vi "test_resist_last.vi"() -> ()   [LabVIEW 2015]
uses:
  global_qaqc.vi
panel:
  out "Output file path":path
  out "Name of PCB":string
  in  "Redo":bool
  out "Last value (MOhm)":dbl
  out "Boolean 16":bool
  out "Boolean 15":bool
  out "Boolean 14":bool
  out "Boolean 13":bool
  out "Boolean 12":bool
  out "Boolean 11":bool
  out "Boolean 10":bool
  out "Boolean 9":bool
  out "Boolean 8":bool
  out "Boolean 7":bool
  out "Boolean 6":bool
  out "Boolean 5":bool
  out "Boolean 4":bool
  out "Boolean 3":bool
  out "Boolean 2":bool
  out "Boolean":bool
  in  "Open Database":bool
  in  "Close VI":bool
  in  "?":bool
  # "Electrometer Test"
  # "1) Setup the measure and then click \"Acquire\". If you want to take again the last measure, click \"Redo last\" and then \"Acquire\""
  # "Yellow: Done"
  # "Green: OK"
  # "Yellow: Done"
  # "Green: OK"
  # "Circular small LED \n\nGREY --> Measure NOT DONE\nYELLOW --> Measure DONE\n\n\nElliptic big LED\n\nRED --> Value not taken OR out of range\nGREEN --> Value in range"
  # "2) Once measure is finished, open the database and upload the file"
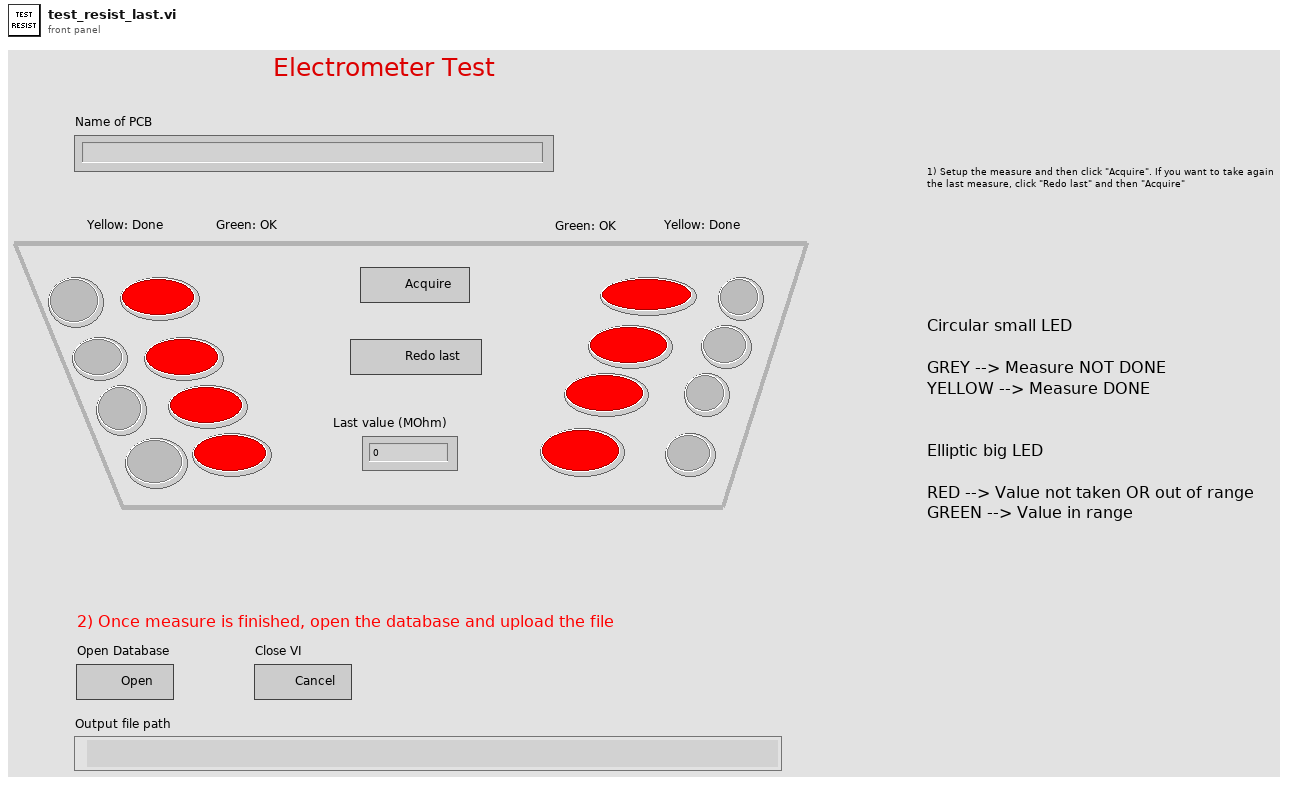
[diagram p1: front panel]
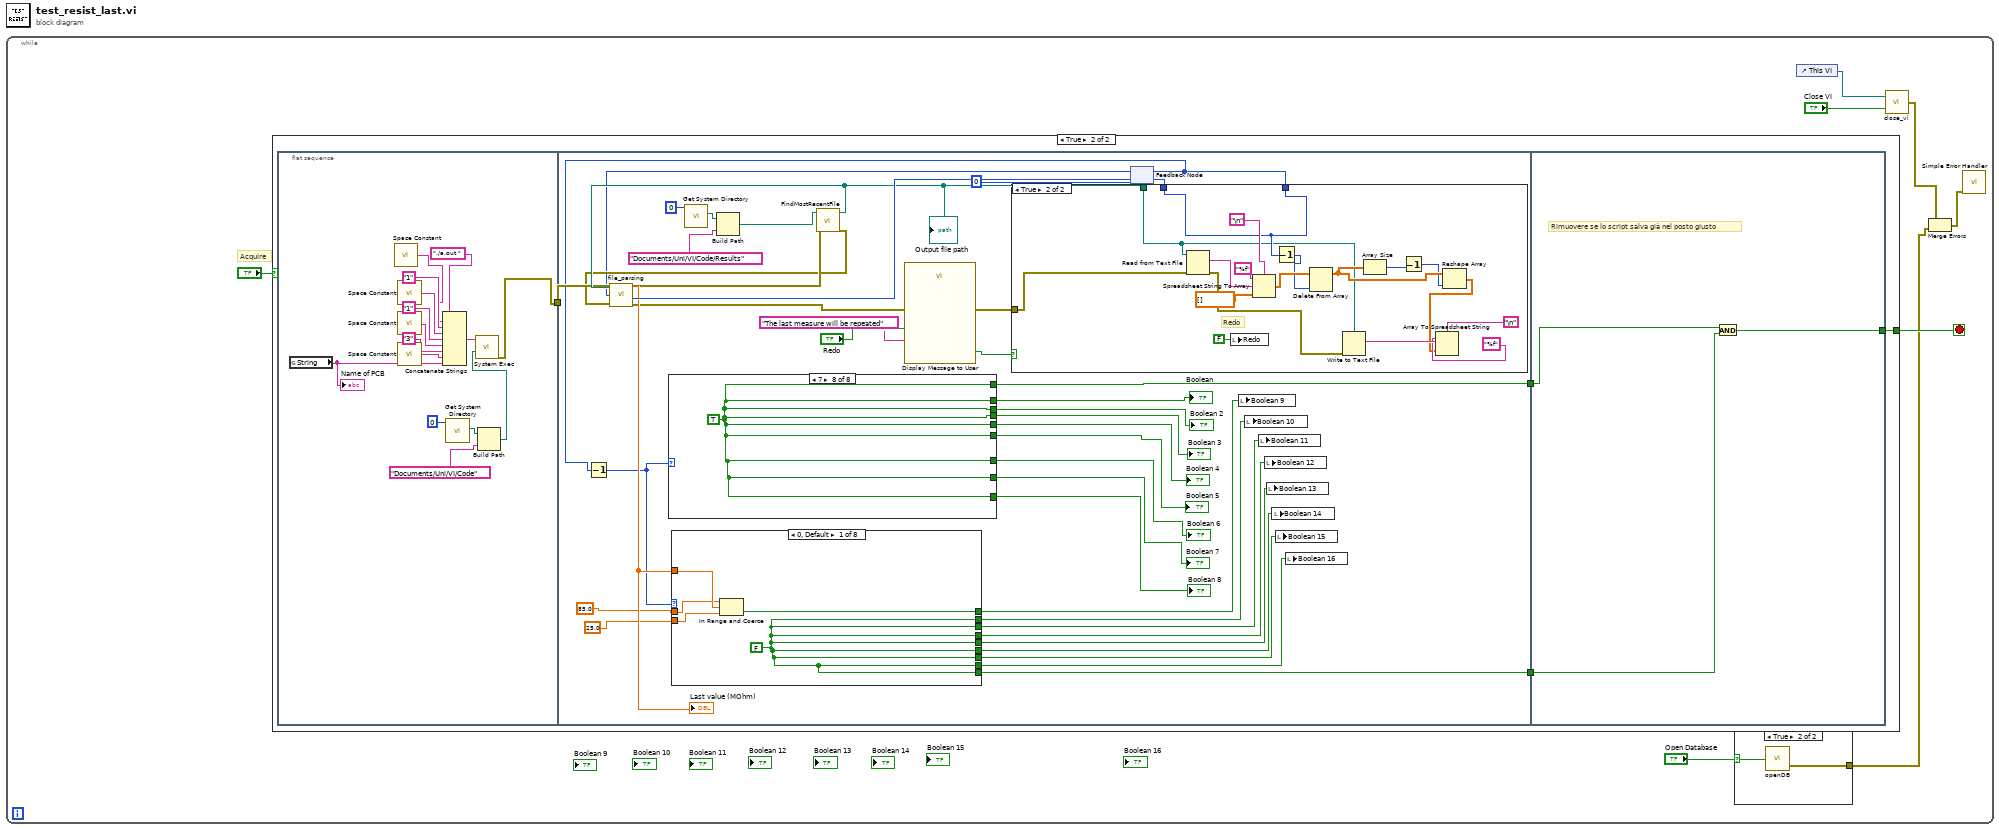
[diagram p0: block diagram]
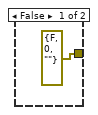
[diagram p2: hidden frame]
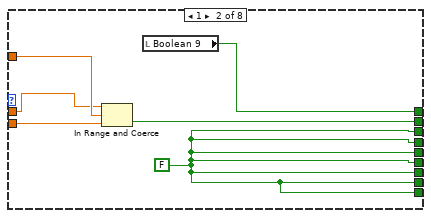
[diagram p4: hidden frame]
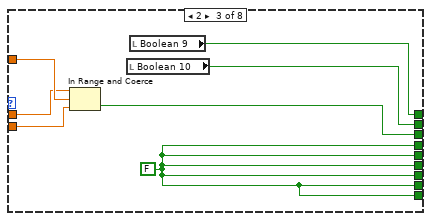
[diagram p5: hidden frame]
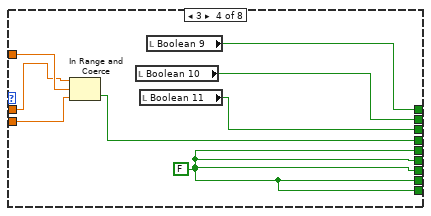
[diagram p6: hidden frame]
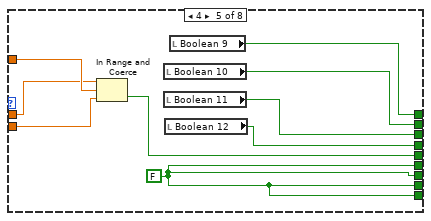
[diagram p7: hidden frame]
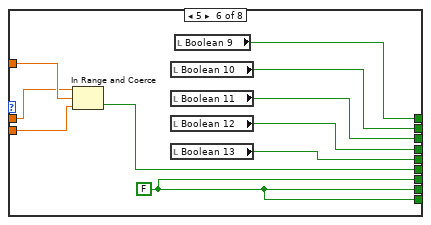
[diagram p8: hidden frame]
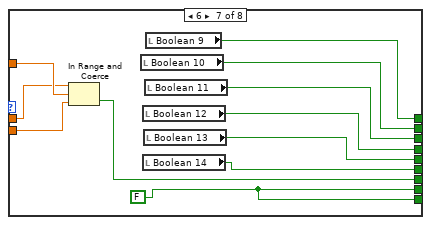
[diagram p9: hidden frame]
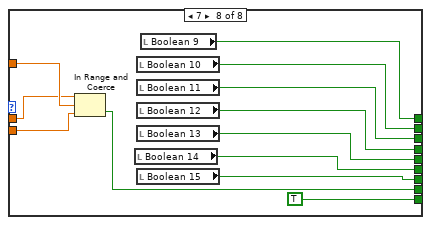
[diagram p10: hidden frame]
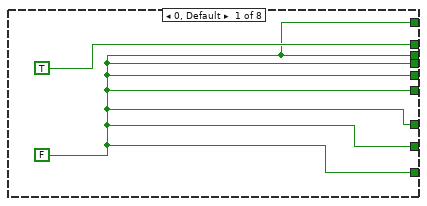
[diagram p11: hidden frame]
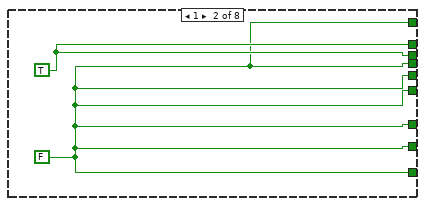
[diagram p12: hidden frame]
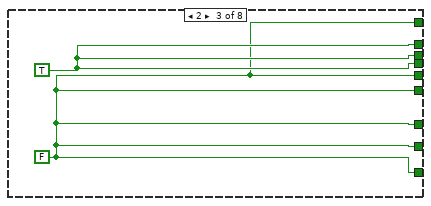
[diagram p13: hidden frame]
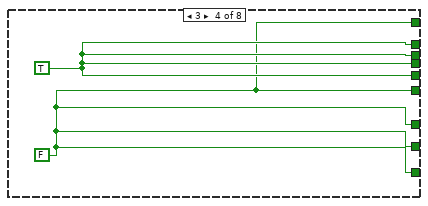
[diagram p14: hidden frame]
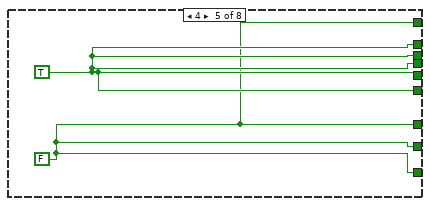
[diagram p15: hidden frame]
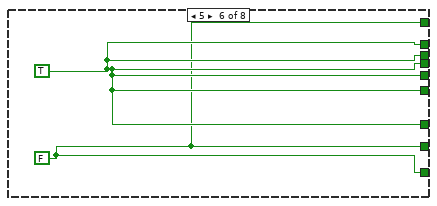
[diagram p16: hidden frame]
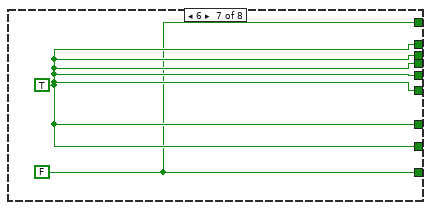
[diagram p17: hidden frame]
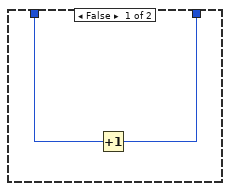
[diagram p18: hidden frame]
diagram:
  n1 = while {
    stop <- w4 stop-if-true
    # "Acquire"
    n2 = case shown="True" "?" {
      selector: "?" -> [w12 _]
      tunnel: [w12 w13] -> w4
      frame False {
      }
      frame True {
        n3 = flat-sequence {
          tunnel: [w17] -> w16
          tunnel: w16 -> [w42]
          tunnel: [w49] -> w15
          tunnel: [w48] -> w14
          tunnel: w15 -> [w174]
          tunnel: w14 -> [w173]
          tunnel: [w172] -> w13
          frame #0 {
            n4 = global read "global_qaqc.vi" "String"() -> (w31:string)
            "Name of PCB" <- w31
            n5 = call <vilib>:"Space Constant.vi"() -> ("String"=w24:string)
            n6 = call <vilib>:"Space Constant.vi"() -> ("String"=w25:string)
            n7 = call <vilib>:"Space Constant.vi"() -> ("String"=w26:string)
            n8 = call <vilib>:"Space Constant.vi"() -> ("String"=w30:string)
            n9 = Concatenate Strings("./a.out " ("String"), w24, "1", w25, "1", w26, "3", w30, w31) -> (w18:string)
            n10 = call <vilib>:"Get System Directory.vi"("system directory type"=0) -> ("system directory"=w21:path)  [unwired: 10 in]
            n11 = Build Path(base path=w21, name or relative path="Documents/Uni/VI/Code") -> (appended path=w19:path)
            n12 = call <vilib>:"System Exec.vi"("working directory"=w19, "command line"=w18) -> ("error out"=w17:errorcluster)  [unwired: 6 in, 3 out]
          }
          frame #1 {
            n13 = call <vilib>:"Get System Directory.vi"("system directory type"=0) -> ("system directory"=w46:path)  [unwired: 10 in]
            n14 = Build Path(base path=w46, name or relative path="Documents/Uni/VI/Code/Results") -> (appended path=w44:path)
            n15 = call "FindMostRecentFile.vi"("error in"=w42, "Folder Path In"=w44) -> ("error out"=w41:errorcluster, "File Path Out"=w43:path)  [unwired: 8 in]
            "Output file path" <- w43
            n16 = call "Display Message to User"("Enable"="Redo", "Message"="The last measure will be repeated") -> ("OK"=w32:bool)  [unwired: 8 in, 1 out]
            n17 = feedback #1(0) -> (w40:i32)
            n18 = call "file_parsing.vi"("File Path Control"=w43, "line index"=w40, "error in"=w41) -> ("Waveform Chart"=w58:dbl, "index output"=w67:i32, "error out"=w35:errorcluster)  [unwired: 1 out]
            "Last value (MOhm)" <- w58
            n19 = case shown="True" w32 {
              tunnel: w67 -> [w153 w156]
              tunnel: [w152 w156] -> w39
              tunnel: w43 -> [_ w155]
              tunnel: w35 -> [_ w154]
              frame False {
                n20 = Increment(x=w153) -> (x+1=w152:i32)
              }
              frame True {
                # "Redo"
                n21 = Read from Text File(file (use dialog)=w155, error in=w154) -> (text=w170:string, error out=w171:errorcluster)  [unwired: 2 in, 2 out]
                n22 = local write "Redo"(FALSE ("redo")) -> ()
                n23 = Spreadsheet String To Array(delimiter (Tab)="\n", format string="%f", spreadsheet string=w170, array type (2D Dbl)=dbl[] []) -> (array=w167:dbl[])
                n24 = Decrement(x=w156) -> (x-1=w157:i32)
                n25 = Delete From Array(array=w167, index=w157) -> (array with subset deleted=w160:dbl[])  [unwired: 1 in, 1 out]
                n26 = Array Size(array=w160) -> (size(s)=w161:i32)
                n27 = Decrement(x=w161) -> (x-1=w159:i32)
                n28 = Reshape Array(w160, w159) -> (w158:dbl[])
                n29 = Array To Spreadsheet String(delimiter (Tab)="\n", array=w158, 3:"%f" ("format string")) -> (spreadsheet string=w165:string)
                n30 = Write to Text File(file (use dialog)=w155, text=w165, error in=w171) -> ()  [unwired: 1 in, 3 out]
              }
            }
            n31 = Decrement(x=w39) -> (x-1=w38:i32)
            n32 = case shown="7" w38 {
              tunnel: [TRUE ("new element/subarray") w140 w142 w144 w146 w148 w150 w151] -> w66
              tunnel: [w137 w140 w142 w144 w146 w148 w150 w151] -> w65
              tunnel: [w137 w139 w142 w144 w146 w148 w150 w151] -> w64
              tunnel: [w137 w139 w141 w144 w146 w148 w150 w151] -> w63
              tunnel: [w137 w139 w141 w143 w146 w148 w150 w151] -> w62
              tunnel: [w137 w139 w141 w143 w145 w148 w150 w151] -> w61
              tunnel: [w137 w139 w141 w143 w145 w147 w150 w151] -> w60
              tunnel: [w137 w139 w141 w143 w145 w147 w149 w151] -> w59
              tunnel: [w137 w139 w141 w143 w145 w147 w149 w151] -> w49
              frame 0, Default {
                w137 = FALSE
              }
              frame 1 {
                w139 = FALSE
                w140 = TRUE ("new element/subarray")
              }
              frame 2 {
                w141 = FALSE
                w142 = TRUE ("new element/subarray")
              }
              frame 3 {
                w143 = FALSE
                w144 = TRUE ("new element/subarray")
              }
              frame 4 {
                w145 = FALSE
                w146 = TRUE ("new element/subarray")
              }
              frame 5 {
                w147 = FALSE
                w148 = TRUE ("new element/subarray")
              }
              frame 6 {
                w149 = FALSE
                w150 = TRUE ("new element/subarray")
              }
              frame 7 {
                w151 = TRUE ("new element/subarray")
              }
            }
            "Boolean 6" <- w61
            "Boolean" <- w66
            "Boolean 3" <- w64
            "Boolean 4" <- w63
            "Boolean 8" <- w59
            "Boolean 2" <- w65
            "Boolean 7" <- w60
            "Boolean 5" <- w62
            n33 = case shown="0, Default" w38 {
              tunnel: w58 -> [w73 w79 w86 w94 w103 w113 w124 w136]
              tunnel: [w71 w77 w84 w91 w100 w110 w121 w133] -> w56
              tunnel: [w71 w76 w83 w90 w99 w109 w120 w132] -> w55
              tunnel: [w71 w76 w82 w93 w98 w108 w119 w131] -> w54
              tunnel: [w71 w76 w82 w89 w102 w107 w118 w130] -> w53
              tunnel: [w71 w76 w82 w89 w97 w112 w117 w129] -> w52
              tunnel: [w71 w76 w82 w89 w97 w106 w123 w128] -> w51
              tunnel: [w71 w76 w82 w89 w97 w106 w116 w135] -> w50
              tunnel: [w72 w78 w85 w92 w101 w111 w122 w134] -> w57
              tunnel: [w71 w76 w82 w89 w97 w106 w116 TRUE] -> w48
              tunnel: 85.0 ("upper limit") -> [w70 w75 w81 w88 w96 w105 w115 w126]
              tunnel: 25.0 ("lower limit") -> [w69 w74 w80 w87 w95 w104 w114 w125]
              frame 0, Default {
                w71 = FALSE
                n34 = In Range and Coerce(upper limit=w70, x=w73, lower limit=w69) -> (In Range?=w72:bool)  [unwired: 1 out]
              }
              frame 1 {
                w76 = FALSE
                n35 = In Range and Coerce(upper limit=w75, x=w79, lower limit=w74) -> (In Range?=w77:bool)  [unwired: 1 out]
                n36 = local read "Boolean 9"() -> (w78:bool)
              }
              frame 2 {
                w82 = FALSE
                n37 = In Range and Coerce(upper limit=w81, x=w86, lower limit=w80) -> (In Range?=w83:bool)  [unwired: 1 out]
                n38 = local read "Boolean 10"() -> (w84:bool)
                n39 = local read "Boolean 9"() -> (w85:bool)
              }
              frame 3 {
                w89 = FALSE
                n40 = In Range and Coerce(upper limit=w88, x=w94, lower limit=w87) -> (In Range?=w93:bool)  [unwired: 1 out]
                n41 = local read "Boolean 10"() -> (w91:bool)
                n42 = local read "Boolean 11"() -> (w90:bool)
                n43 = local read "Boolean 9"() -> (w92:bool)
              }
              frame 4 {
                w97 = FALSE
                n44 = In Range and Coerce(upper limit=w96, x=w103, lower limit=w95) -> (In Range?=w102:bool)  [unwired: 1 out]
                n45 = local read "Boolean 10"() -> (w100:bool)
                n46 = local read "Boolean 11"() -> (w99:bool)
                n47 = local read "Boolean 12"() -> (w98:bool)
                n48 = local read "Boolean 9"() -> (w101:bool)
              }
              frame 5 {
                w106 = FALSE
                n49 = In Range and Coerce(upper limit=w105, x=w113, lower limit=w104) -> (In Range?=w112:bool)  [unwired: 1 out]
                n50 = local read "Boolean 10"() -> (w110:bool)
                n51 = local read "Boolean 11"() -> (w109:bool)
                n52 = local read "Boolean 12"() -> (w108:bool)
                n53 = local read "Boolean 13"() -> (w107:bool)
                n54 = local read "Boolean 9"() -> (w111:bool)
              }
              frame 6 {
                w116 = FALSE
                n55 = In Range and Coerce(upper limit=w115, x=w124, lower limit=w114) -> (In Range?=w123:bool)  [unwired: 1 out]
                n56 = local read "Boolean 10"() -> (w121:bool)
                n57 = local read "Boolean 12"() -> (w119:bool)
                n58 = local read "Boolean 14"() -> (w117:bool)
                n59 = local read "Boolean 13"() -> (w118:bool)
                n60 = local read "Boolean 11"() -> (w120:bool)
                n61 = local read "Boolean 9"() -> (w122:bool)
              }
              frame 7 {
                n62 = In Range and Coerce(upper limit=w126, x=w136, lower limit=w125) -> (In Range?=w135:bool)  [unwired: 1 out]
                n63 = local read "Boolean 14"() -> (w129:bool)
                n64 = local read "Boolean 10"() -> (w133:bool)
                n65 = local read "Boolean 11"() -> (w132:bool)
                n66 = local read "Boolean 12"() -> (w131:bool)
                n67 = local read "Boolean 13"() -> (w130:bool)
                n68 = local read "Boolean 15"() -> (w128:bool)
                n69 = local read "Boolean 9"() -> (w134:bool)
              }
            }
            n70 = feedback-in #1(w39) -> ()
            n71 = local write "Boolean 9"(w57) -> ()
            n72 = local write "Boolean 10"(w56) -> ()
            n73 = local write "Boolean 11"(w55) -> ()
            n74 = local write "Boolean 12"(w54) -> ()
            n75 = local write "Boolean 13"(w53) -> ()
            n76 = local write "Boolean 14"(w52) -> ()
            n77 = local write "Boolean 15"(w51) -> ()
            n78 = local write "Boolean 16"(w50) -> ()
          }
          frame #2 {
            # "Rimuovere se lo script salva già nel posto giusto"
            n79 = And(x=w174, y=w173) -> (x .and. y?=w172:bool)
          }
        }
      }
    }
    n80 = case shown="True" "Open Database" {
      selector: "Open Database" -> [_ w11]
      tunnel: [errorcluster {"status"=FALSE, "code"=0, "source"=""} ("error out") w10] -> w1
      frame False {
      }
      frame True {
        n81 = call "openDB.vi"("Open Button"=w11) -> ("error out"=w10:errorcluster)  [unwired: 1 out]
      }
    }
    n82 = control-ref of="This VI"() -> (w6:refnum<vi>)
    n83 = call "close_vi.vi"("Process Stop Button"="Close VI", "reference"=w6) -> ("error out"=w3:errorcluster)
    n84 = Merge Errors(w3, w1) -> (w2:errorcluster)
    n85 = call <vilib>:"Simple Error Handler.vi"("error in (no error)"=w2) -> ()  [unwired: 4 in, 5 out]
  }
